vi "Read Path type.vi"(8 "error in (no error)":errorcluster, 11 "Load-file in":refnum<class "Load-file.lvclass">) -> (0 "error out":errorcluster, 2 "Path type":bool, 3 "Load-file out":refnum<class "Load-file.lvclass">)   [LabVIEW 2013, in "Messages.lvlib" / "Load-file.lvclass"]
uses:
  Load-file.lvclass
  Load-file.lvclass/Load-file.ctl
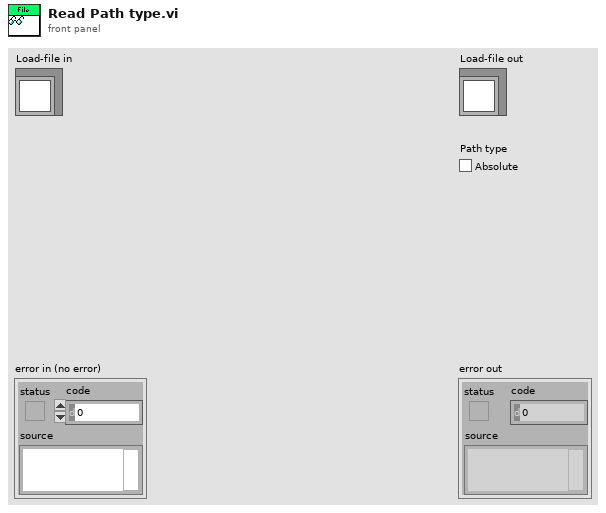
[diagram p1: front panel]
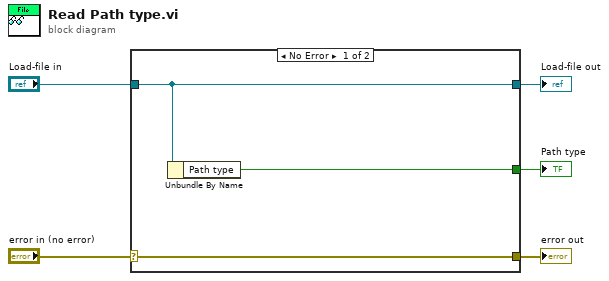
[diagram p0: block diagram]
diagram:
  n1 = case shown="No Error" "error in (no error)" {
    selector: "error in (no error)" -> [w8 w9]
    tunnel: [w8 w9] -> w4
    tunnel: [w7 w10] -> w2
    tunnel: "Load-file in" -> [w7 w10]
    tunnel: [w6 _] -> w1
    frame No Error {
      n2 = Unbundle By Name(w7) -> ("Path type"=w6:bool)
    }
    frame Error {
    }
  }
  "error out" <- w4
  "Load-file out" <- w2
  "Path type" <- w1
